vi "XPert Phone Modem Connect.vi"() -> ()   [LabVIEW 2016]
uses:
  <vilib>/Instr/_visa.llb/VISA Configure Serial Port (Instr).vi
panel:
  out "read buffer 2":string
  in  "baud rate (9600)":u32=9600
  out "read buffer":string
  out "error out":errorcluster
  in  "error in (no error)":errorcluster
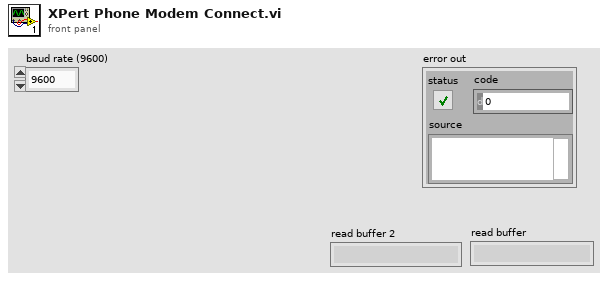
[diagram p1: front panel]
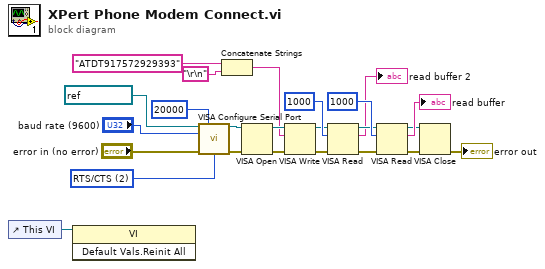
[diagram p0: block diagram]
diagram:
  w12 = u16 2 items=["None", "XON/XOFF", "RTS/CTS", "XON/XOFF & RTS/CTS", "DTR/DSR", "XON/XOFF & DTR/DSR"] ("flow control (0:none)")
  n1 = control-ref of="This VI"() -> (w1:refnum<vi>)
  n2 = invoke class="VI" method="Default Vals.Reinit All"(reference=w1) -> ()  [unwired: 2 in, 3 out]
  n3 = call-poly "VISA Configure Serial Port"("VISA resource name"=refnum<visa-resource-name> "COM16", "timeout (10sec)"=u32 20000, "baud rate (9600)"="baud rate (9600)", "error in (no error)"="error in (no error)", "flow control (0:none)"=w12) -> ("VISA resource name out"=w16:refnum<visa-resource-name>, "error out"=w17:errorcluster)  [unwired: 9 in]
  n4 = Concatenate Strings("ATDT917572929393" ("string"), "\r\n") -> (w9:string)
  n5 = VISA Open(error in (no error)=w17, VISA resource name=w16) -> (VISA resource name=w19:refnum<visa-resource-name>, error out=w20:errorcluster)  [unwired: 3 in]
  n6 = VISA Write(VISA resource name=w19, write buffer=w9, error in (no error)=w20) -> (VISA resource name out=w14:refnum<visa-resource-name>, error out=w13:errorcluster)  [unwired: 1 out]
  n7 = VISA Read(VISA resource name=w14, byte count=u32 1000, error in (no error)=w13) -> (VISA resource name out=w7:refnum<visa-resource-name>, read buffer=→"read buffer 2":string, error out=w5:errorcluster)  [unwired: 1 out]
  n8 = VISA Read(VISA resource name=w7, byte count=u32 1000, error in (no error)=w5) -> (VISA resource name out=w4:refnum<visa-resource-name>, read buffer=→"read buffer":string, error out=w3:errorcluster)  [unwired: 1 out]
  n9 = VISA Close(VISA resource name=w4, error in (no error)=w3) -> (error out=→"error out":errorcluster)
